vi "Terminal_Drive_Syetem_Display.vi"   [LabVIEW 2014]
types:
  T1 = cluster{"变送器配电模块电压":u16, "变频器电流":u16, "变频器电压":u16, "变频器频率":u16, "动力子系统状态字":cluster{"电机温度过高报警":bool, "变频器电气参数异常报警":bool, "电机过载报警":bool, "电机转速误差过大报警":bool}}
  T2 = cluster{"变送器配电模块电压":u16, "变频器电流":u16, "变频器电压":u16, "变频器频率":u16}
  T3 = cluster{"电机温度过高报警":bool, "变频器电气参数异常报警":bool, "电机过载报警":bool, "电机转速误差过大报警":bool}
  T4 = cluster{cluster{sgl, sgl, "变送器配电模块电压":u16}, cluster{sgl, sgl, "变频器电流":u16}, cluster{sgl, sgl, "变频器电压":u16}, cluster{sgl, sgl, "变频器频率":u16}, "动力子系统状态字":cluster{"电机温度过高报警":bool, "变频器电气参数异常报警":bool, "电机过载报警":bool, "电机转速误差过大报警":bool}}
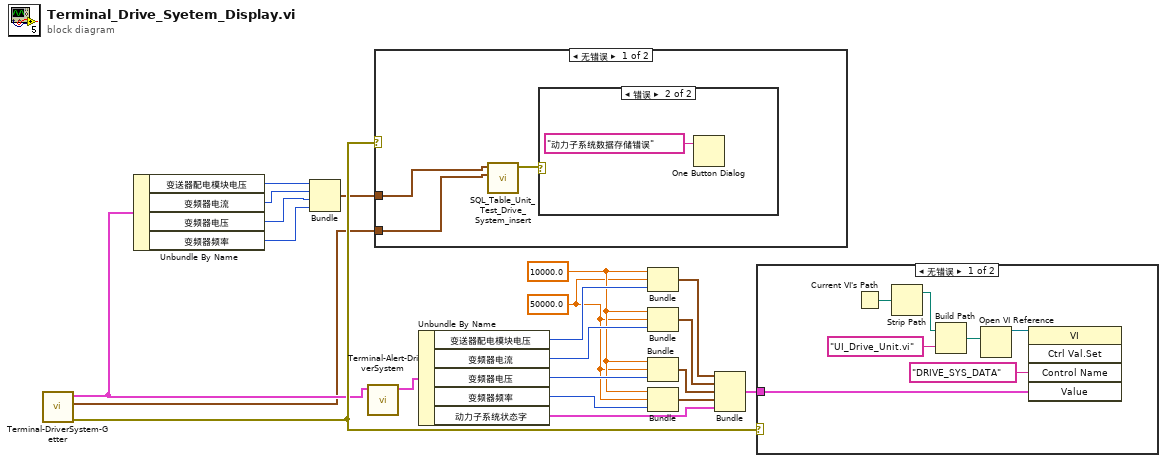
[diagram p0: block diagram]
diagram:
  w16 = sgl 50000.0
  w17 = sgl 10000.0
  n1 = call "Terminal-DriverSystem-Getter.vi"() -> ("error out"=w8:errorcluster, "时间标识"=w1:timestamp, "设备信息"=w7:T1)  [unwired: 9 in]
  n2 = Unbundle By Name(w7) -> ("变送器配电模块电压"=w6:u16, "变频器电流"=w5:u16, "变频器电压"=w4:u16, "变频器频率"=w3:u16)
  n3 = Bundle("变送器配电模块电压"=w6, "变频器电流"=w5, "变频器电压"=w4, "变频器频率"=w3) -> (w2:T2)  [unwired: 1 in]
  n4 = call "Terminal-Alert-DriverSystem.vi"("动力子系统设备信息"=w7) -> ("动力子系统设备信息输出"=w9:T1)  [unwired: 10 in]
  n5 = case shown="无错误" w8 {
    tunnel: w2 -> [w24 _]
    tunnel: w1 -> [w23 _]
    frame No Error {
      n6 = call "SQL_Table_Unit_Test_Drive_System_insert.vi"("时间标识"=w23, "动力子系统数据"=w24) -> ("error out"=w22:errorcluster)  [unwired: 9 in]
      n7 = case shown="错误" w22 {
        frame No Error {
        }
        frame Error {
          n8 = One Button Dialog(message="动力子系统数据存储错误" ("消息")) -> ()  [unwired: 1 in, 1 out]
        }
      }
    }
    frame Error {
    }
  }
  n9 = Unbundle By Name(w9) -> ("变送器配电模块电压"=w21:u16, "变频器电流"=w20:u16, "变频器电压"=w19:u16, "变频器频率"=w18:u16, "动力子系统状态字"=w11:T3)
  n10 = Bundle(w17, w16, "变送器配电模块电压"=w21) -> (w15:cluster{sgl, sgl, "变送器配电模块电压":u16})  [unwired: 1 in]
  n11 = Bundle(w17, w16, "变频器电流"=w20) -> (w14:cluster{sgl, sgl, "变频器电流":u16})  [unwired: 1 in]
  n12 = Bundle(w17, w16, "变频器电压"=w19) -> (w13:cluster{sgl, sgl, "变频器电压":u16})  [unwired: 1 in]
  n13 = Bundle(w17, w16, "变频器频率"=w18) -> (w12:cluster{sgl, sgl, "变频器频率":u16})  [unwired: 1 in]
  n14 = Bundle(w15, w14, w13, w12, "动力子系统状态字"=w11) -> (w10:T4)  [unwired: 1 in]
  n15 = case shown="无错误" w8 {
    tunnel: w10 -> [w26 _]
    frame No Error {
      n16 = Current VI's Path() -> (path=w30:path)
      n17 = Strip Path(path=w30) -> (stripped path=w31:path)  [unwired: 1 out]
      n18 = Build Path(base path=w31, name or relative path="UI_Drive_Unit.vi") -> (appended path=w28:path)
      n19 = Open VI Reference(vi path=w28) -> (vi reference=w27:refnum<vi>)  [unwired: 5 in, 1 out]
      n20 = invoke class="VI" method="Ctrl Val.Set"(reference=w27, "Control Name"="DRIVE_SYS_DATA", "Value"=w26) -> ()  [unwired: 2 in, 5 out]
    }
    frame Error {
    }
  }
